vi "Add Data Set to Running Mean.vi"(10 "JSON Data Set":refnum<class "JSON Value.lvclass">, 11 "Statistics in":refnum<class "JSON Value.lvclass">) -> (3 "Statistics":refnum<class "JSON Value.lvclass">)   [LabVIEW 2020, in "Library Commun.lvlib" / "JSON Running Mean.lvclass"]
uses:
  JSON Running Mean.lvclass
  JSON Value/JSON Value.lvclass
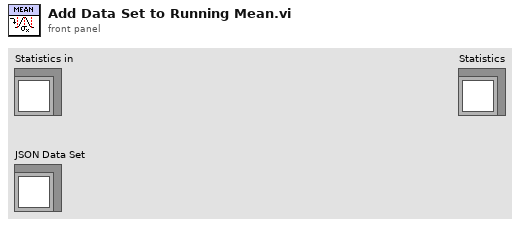
[diagram p1: front panel]
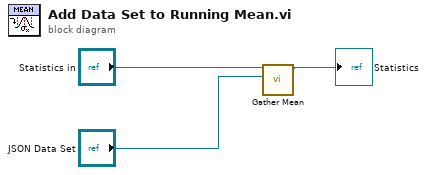
[diagram p0: block diagram]
diagram:
  n1 = call-dynamic "Gather Mean.vi"("JSON Value"="JSON Data Set", "Statistics in"="Statistics in") -> ("Statistics out"=→"Statistics":refnum<class "JSON Value.lvclass">)  [unwired: 9 in]
